vi "Get All KeySight ENA Sessions.vi"(8 "error in (no error)":errorcluster, 11 "Semiconductor Module Context":T1) -> (0 "error out":errorcluster, 2 "Instrument Sessions":refnum<k15>[](array[refnum]), 3 "Semiconductor Module Context Out":T1)   [LabVIEW 2013, in "ENA Custom Instrument.lvlib"]
uses:
  ENA Custom Instrument.lvlib
  <vilib>/NI_TestStand_SemiconductorModule/NI_TestStand_Semiconductor_Module.lvlibp/PinMap/General/SemiconductorModuleContext.ctl
  <vilib>/NI_TestStand_SemiconductorModule/NI_TestStand_Semiconductor_Module.lvlibp
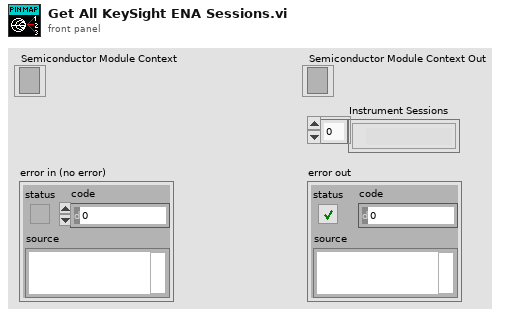
[diagram p1: front panel]
types:
  T1 = typedef "NI_TestStand_Semiconductor_Module.lvlibp/SemiconductorModuleContext.ctl" = refnum<k7>
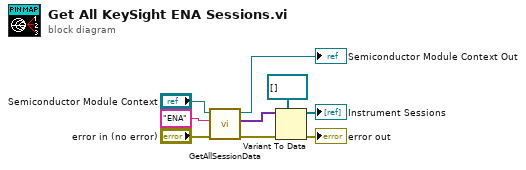
[diagram p0: block diagram]
diagram:
  n1 = call <vilib>:"GetAllSessionData.vi"("error in (no error)"="error in (no error)", "Instrument Type Id"="ENA", "Semiconductor Module Context"="Semiconductor Module Context") -> ("error out"=w5:errorcluster, "Session Data"=w4:variant[], "Semiconductor Module Context Out"=→"Semiconductor Module Context Out":T1)  [unwired: 4 in, 2 out]
  n2 = Variant To Data(error in=w5, type=refnum<k15>[] [], Variant=w4) -> (data=→"Instrument Sessions":refnum<k15>[], error out=→"error out":errorcluster)
